vi "Measure.vi"(8 "error in (no error)":errorcluster, 11 "RMX4120 in":refnum<class "RMX4120.lvclass">) -> (0 "error out":errorcluster, 1 "Current":dbl, 2 "Voltage":dbl, 3 "RMX4120 out":refnum<class "RMX4120.lvclass">, 4 "Power":dbl)   [LabVIEW 2023, in "RMX4120.lvclass"]
uses:
  RMX4120.lvclass
  RMX4120.lvclass/RMX4120.ctl
  RMXPowerSupply.lvclass
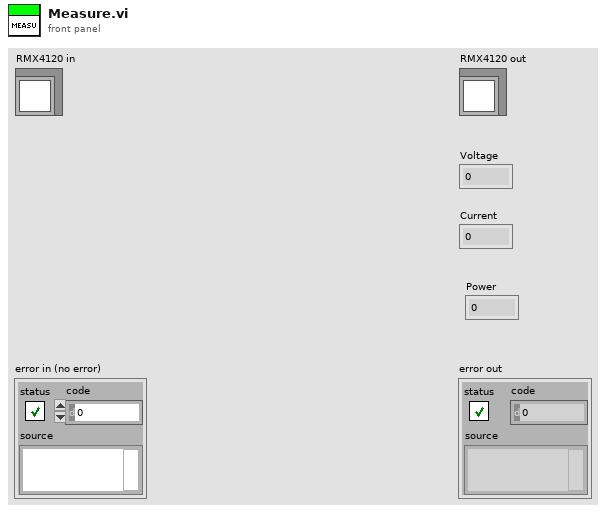
[diagram p1: front panel]
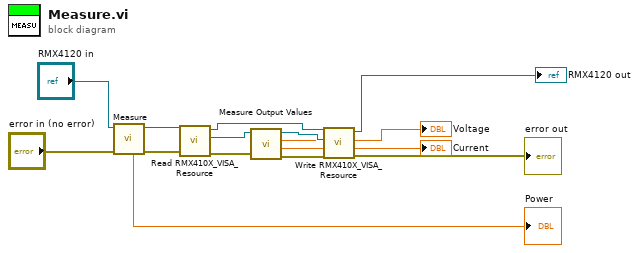
[diagram p0: block diagram]
diagram:
  n1 = call-parent "Measure.vi"("error in (no error)"="error in (no error)", "RMXPowerSupply in"="RMX4120 in") -> ("error out"=w10:errorcluster, "RMXPowerSupply out"=w11:refnum<class "RMX4120.lvclass">, "Power"=→"Power":dbl)  [unwired: 5 in, 2 out]
  n2 = call-dynamic "Read RMX410X_VISA_Resource.vi"("error in (no error)"=w10, "RMXPowerSupply in"=w11) -> ("error out"=w8:errorcluster, "RMX410X_VISA_Resource"=w9:refnum<visa-resource-name>, "RMXPowerSupply out"=w6:refnum<class "RMX4120.lvclass">)  [unwired: 7 in]
  n3 = call "Measure Output Values.vi"("error in (no error)"=w8, "VISA resource name"=w9) -> ("error out"=w7:errorcluster, "Current Output"=→"Current":dbl, "Voltage Output"=→"Voltage":dbl, "VISA resource name out"=w3:refnum<visa-resource-name>)  [unwired: 6 in]
  n4 = call-dynamic "Write RMX410X_VISA_Resource.vi"("error in (no error)"=w7, "RMX410X_VISA_Resource"=w3, "RMXPowerSupply in"=w6) -> ("error out"=→"error out":errorcluster, "RMXPowerSupply out"=→"RMX4120 out":refnum<class "RMX4120.lvclass">)  [unwired: 7 in]
